vi "MB Serial Example Master.vi"() -> ()   [LabVIEW 2011]
uses:
  MB Serial Master Query Read Discrete Inputs (poly).vi
  MB Serial Master Query Read Input Registers (poly).vi
  MB Serial Master Query Write Multiple Registers (poly).vi
  MB Serial Master Query Write Multiple Coils (poly).vi
panel:
  in  "Serial Parameters":T1={"Mode"=enum."RTU", "Slave Address"=1}
  in  "Timeout":u32=10000
  in  "Flow Control":u16(ring) items=["None", "XON/XOFF", "RTS/CTS", "XON/XOFF & RTS/CTS", "DTR/DSR", "XON/XOFF & DTR/DSR"]
  in  "Parity":u16(ring) items=["None", "Odd", "Even", "Mark", "Space"]
  in  "Baud Rate":u32=9600
  in  "VISA resource name":refnum<visa-resource-name>
  in  "Stop":bool
  out "Slave Input Registers":u16[](array[numeric]) caption="Slave Input Registers (Read Only)"
  out "Slave Discrete Inputs":bool[](array[boolean])
  in  "Coils to Write":bool[](array[boolean])=[FALSE, FALSE, FALSE, FALSE]
  in  "Registers to Write":u16[](array[numeric])=[0, 0, 0, 0]
  # "MB Serial Example Master.vi\n\nInstructions\n1. Connect your 2 COMs ports using a cross-over cable\n2. Select a COM port in VISA resouce name\n3. Open and run MB Example Slave.vi\n4. Run this VI.\n5. Modify the discrete inputs or input registers on the slave -> they're updated on the master.\n6. Modify the coils and registers on the master -> they're updated on the slave."
  # "Serial Parameters"
  # "Data to write to the slave"
  # "Slave Read-only Registers"
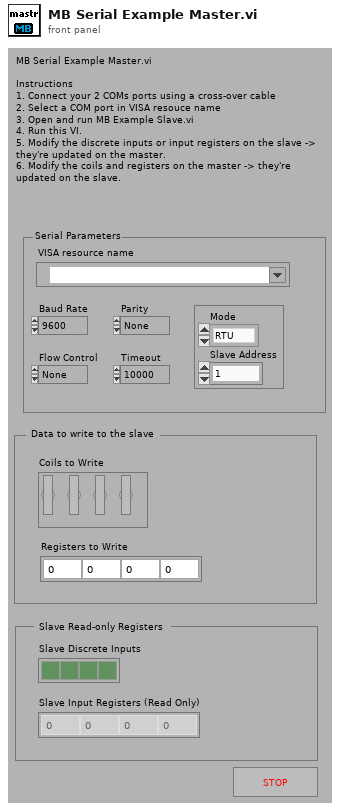
[diagram p1: front panel]
types:
  T1 = cluster{"Mode":enum16{"RTU", "ASCII"}, "Slave Address":u8}
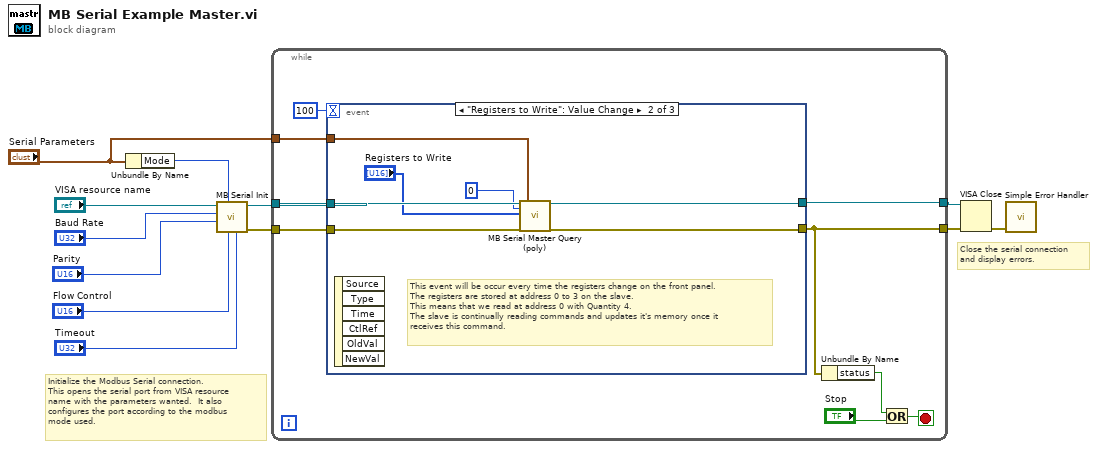
[diagram p0: block diagram]
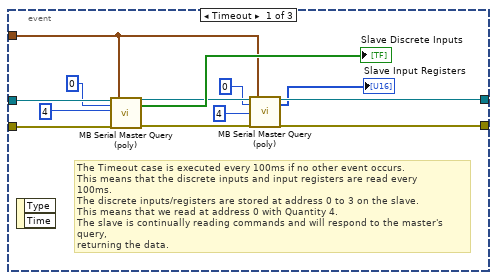
[diagram p2: hidden frame]
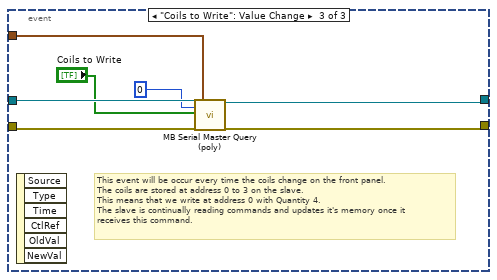
[diagram p3: hidden frame]
diagram:
  # "Close the serial connection\nand display errors."
  # "Initialize the Modbus Serial connection.\nThis opens the serial port from VISA resource\nname with the parameters wanted.  It also\nconfigures the port according to the modbus\nmode used."
  n1 = Unbundle By Name("Serial Parameters") -> ("Mode"=w6:enum16{"RTU", "ASCII"})
  n2 = call "MB Serial Init.vi"("Timeout"="Timeout", "Flow Control"="Flow Control", "Mode"=w6, "Parity"="Parity", "Baud Rate"="Baud Rate", "VISA resource name"="VISA resource name") -> ("error out"=w5:errorcluster, "VISA resource name out"=w11:refnum<visa-resource-name>)  [unwired: 1 in, 3 out]
  n3 = while {
    tunnel: w11 -> [w21]
    tunnel: w5 -> [w20]
    tunnel: "Serial Parameters" -> [w19]
    tunnel: [w15] -> w3
    tunnel: [w14] -> w2
    stop <- w18 stop-if-true
    n4 = event shown="[1] \"Registers to Write\": Value Change" {
      selector: _ -> [_ _ _]
      dyn-events: _ -> [_ _ _]
      timeout: 100 -> [_ _ _]
      tunnel: w21 -> [w34 w41 w48]
      tunnel: w20 -> [w31 w40 w47]
      tunnel: w19 -> [w28 w39 w46]
      tunnel: [w26 w37 w42] -> w14
      tunnel: [w25 w36 w43] -> w15
      event Timeout {
        # "The Timeout case is executed every 100ms if no other event occurs.\nThis means that the discrete inputs and input registers are read every \n100ms.\nThe discrete inputs/registers are stored at address 0 to 3 on the slave.\nThis means that we read at address 0 with Quantity 4.\nThe slave is continually reading commands and will respond to the master's query,\nreturning the data."
        n5 = event-data() -> ()  [unwired: 3 out]
        n6 = call-poly "MB Serial Master Query (poly).vi"("VISA resource name"=w34, "Starting Address"=u16 0, "Quantity"=u16 4, "error in"=w31, "Serial Parameters"=w28) -> ("VISA resource name out"=w29:refnum<visa-resource-name>, "Discrete Inputs"=→"Slave Discrete Inputs":bool[], "error out"=w27:errorcluster)  [unwired: 1 in, 11 out]
        n7 = call-poly "MB Serial Master Query (poly).vi"("VISA resource name"=w29, "Starting Address"=u16 0, "Quantity"=u16 4, "error in"=w27, "Serial Parameters"=w28) -> ("VISA resource name out"=w25:refnum<visa-resource-name>, "Input Registers"=→"Slave Input Registers":u16[], "error out"=w26:errorcluster)  [unwired: 1 in, 11 out]
      }
      event "Registers to Write": Value Change {
        # "This event will be occur every time the registers change on the front panel.\nThe registers are stored at address 0 to 3 on the slave.\nThis means that we read at address 0 with Quantity 4.\nThe slave is continually reading commands and updates it's memory once it\nreceives this command."
        n8 = event-data() -> ()  [unwired: 7 out]
        n9 = call-poly "MB Serial Master Query (poly).vi"("VISA resource name"=w41, "Starting Address"=u16 0, "Registers"="Registers to Write", "error in"=w40, "Serial Parameters"=w39) -> ("VISA resource name out"=w36:refnum<visa-resource-name>, "error out"=w37:errorcluster)  [unwired: 2 in, 11 out]
      }
      event "Coils to Write": Value Change {
        # "This event will be occur every time the coils change on the front panel.\nThe coils are stored at address 0 to 3 on the slave.\nThis means that we write at address 0 with Quantity 4.\nThe slave is continually reading commands and updates it's memory once it\nreceives this command."
        n10 = event-data() -> ()  [unwired: 7 out]
        n11 = call-poly "MB Serial Master Query (poly).vi"("VISA resource name"=w48, "Starting Address"=u16 0, "Coils"="Coils to Write", "error in"=w47, "Serial Parameters"=w46) -> ("VISA resource name out"=w43:refnum<visa-resource-name>, "error out"=w42:errorcluster)  [unwired: 2 in, 11 out]
      }
    }
    n12 = Unbundle By Name(w14) -> ("status"=w16:bool)
    n13 = Or(x=w16, y="Stop") -> (x .or. y?=w18:bool)
  }
  n14 = VISA Close(VISA resource name=w3, error in (no error)=w2) -> (error out=w1:errorcluster)
  n15 = call <vilib>:"Simple Error Handler.vi"("error in (no error)"=w1) -> ()  [unwired: 1 in, 8 out]
